vi "arduino sensirion read to stream and log (sub-vi).vi"(0 "logfile refnum":refnum<file>, 1 "VISA resource name (COM3)":refnum<visa-resource-name>="COM3", 2 "stop channel":T1, 5 "read byte count (512)":u32=512, 7 "expected num sensors (12)":i32=12, 9 "baud rate (576000)":u32=576000, 11 "error in (no error)":errorcluster) -> (8 "sensor data cluster channel":T2, 15 "error out":errorcluster)   [LabVIEW 2021]
uses:
  <extravilib>/ChannelInstances/Stream-t'sensirion_data_with_time.ctl'/)Channel.ctl
  type-defs/sensirion_data_with_time.ctl
  controls/sensirion_flow_sensor_data.ctl
  <extravilib>/ChannelInstances/Tag-bool/))Channel.ctl
  <extravilib>/ChannelInstances/Stream-t'sensirion_data_with_time.ctl'/Read With Abort.vi
  <extravilib>/ChannelInstances/Stream-t'sensirion_data_with_time.ctl'/Write With Abort.vi
  <extravilib>/ChannelInstances/Stream-t'sensirion_data_with_time.ctl'/EndpointRead.vi
  <extravilib>/ChannelInstances/Tag-bool/Read With Abort.vi
  <extravilib>/ChannelInstances/Tag-bool/Write With Abort.vi
  <extravilib>/ChannelInstances/Stream-t'sensirion_data_with_time.ctl'/Endpoint.vi
  <vilib>/Instr/_visa.llb/VISA Configure Serial Port (Instr).vi
  <extravilib>/ChannelInstances/Tag-bool/Instantiate.vi
  <extravilib>/ChannelInstances/Stream-t'sensirion_data_with_time.ctl'/Instantiate.vi
  <extravilib>/ChannelInstances/Stream-t'sensirion_data_with_time.ctl'/)Channel.vi
  <resource>/ChannelSupport/_ChannelSupport/WaitIfNeeded.vi
  <extravilib>/ChannelInstances/Tag-bool/EndpointRead.vi
  <extravilib>/ChannelInstances/Tag-bool/Endpoint.vi
  <extravilib>/ChannelInstances/Stream-t'sensirion_data_with_time.ctl'.lvlib
  <extravilib>/ChannelInstances/Tag-bool.lvlib
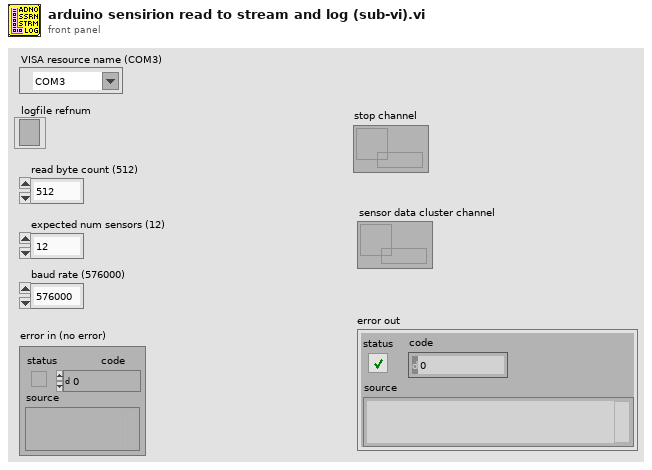
[diagram p1: front panel]
types:
  T1 = typedef "Tag-bool.lvlib/))Channel.ctl" = refnum<queue>
  T2 = typedef "Stream-t'sensirion_data_with_time.ctl'.lvlib/)Channel.ctl" = refnum<queue>
  T3 = typedef "sensirion_data_with_time.ctl" = cluster{"sensor data array":T4[], "relative timestamp":dbl, "error":errorcluster}
  T4 = typedef "sensirion_flow_sensor_data.ctl" = cluster{"flow rate \n":dbl[unit], "flow val. status":bool, "temperature":dbl[unit], "temp. val status":bool, "air in line?":bool, "high flow?":bool, "flag. val status":bool}
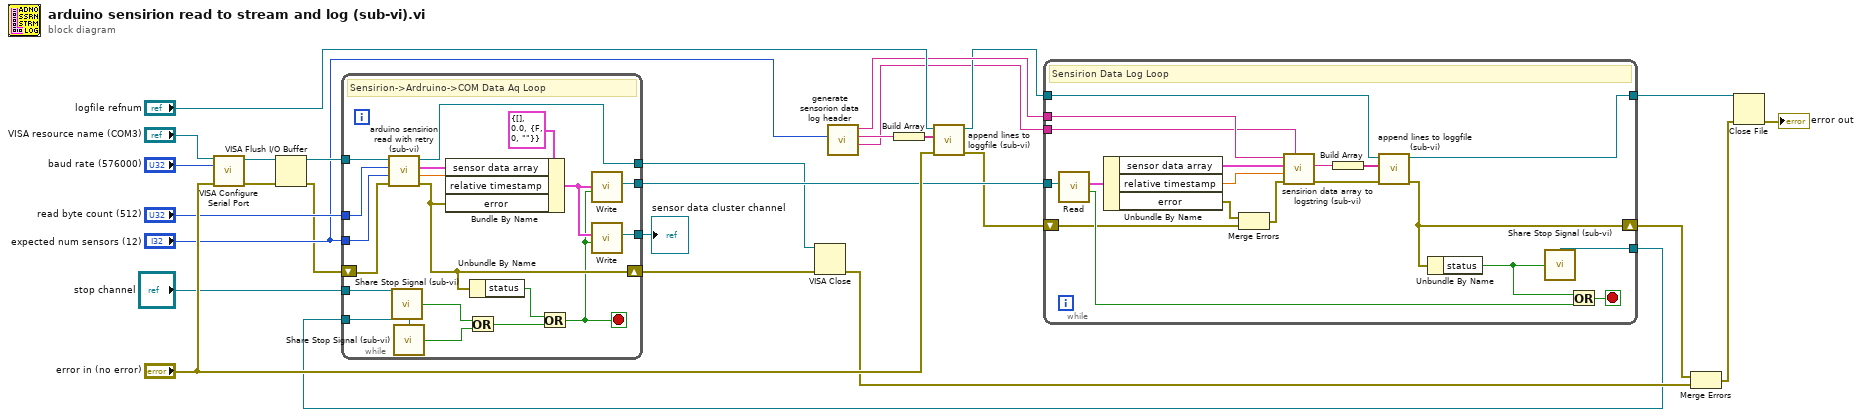
[diagram p0: block diagram]
diagram:
  n1 = call-poly "VISA Configure Serial Port"("VISA resource name"="VISA resource name (COM3)", "baud rate (9600)"="baud rate (576000)", "error in (no error)"="error in (no error)") -> ("VISA resource name out"=w23:refnum<visa-resource-name>, "error out"=w22:errorcluster)  [unwired: 11 in]
  n2 = VISA Flush I/O Buffer(VISA resource name=w23, error in (no error)=w22) -> (VISA resource name out=w18:refnum<visa-resource-name>, error out=w13:errorcluster)  [unwired: 1 in]
  n3 = call "generate sensorion data log header.vi"("num sensors"="expected num sensors (12)") -> ("delimiter"=w6:string, "sensor data header string"=w21:string, "value format"=w14:string)  [unwired: 8 in]
  n4 = Build Array(w21) -> (w20:string[])
  n5 = call "append lines to loggfile (sub-vi).vi"("error in (no error)"="error in (no error)", "string array"=w20, "file refnum"="logfile refnum") -> ("error out"=w9:errorcluster, "file refnum out"=w12:refnum<file>)  [unwired: 7 in]
  n6 = while {
    tunnel: "read byte count (512)" -> [w46]
    tunnel: w18 -> [w45]
    tunnel: [w39] -> w17
    tunnel: "expected num sensors (12)" -> [w38]
    shift-right: [w35] -> w5
    shift-left: w13 -> [w44]
    tunnel: [w37] -> w11
    tunnel: "stop channel" -> [w36]
    tunnel: [w32] -> w3
    tunnel: w1 -> [w31]
    stop <- w33 stop-if-true
    # "Sensirion->Ardruino->COM Data Aq Loop"
    n7 = call "arduino sensirion read with retry (sub-vi).vi"("error in (no error)"=w44, "expected num sensors (12)"=w38, "read byte count (512)"=w46, "VISA resource name"=w45) -> ("error out"=w35:errorcluster, "relative timestamp"=w41:dbl, "sensor data array"=w42:T4[], "VISA resource name out"=w32:refnum<visa-resource-name>)  [unwired: 3 in, 1 out]
    n8 = call "Share Stop Signal (sub-vi).vi"("channel"=w36) -> ("stop"=w30:bool)  [unwired: 1 in]
    n9 = call "Share Stop Signal (sub-vi).vi"("channel"=w31) -> ("stop"=w28:bool)  [unwired: 1 in]
    n10 = Bundle By Name(cluster=T3 {"sensor data array"=[], "relative timestamp"=0.0, "error"={"status"=FALSE, "code"=0, "source"=""}} ("Cluster"), "sensor data array"=w42, "relative timestamp"=w41, "error"=w35) -> (w40:T3)
    n11 = Or(x=w30, y=w28) -> (x .or. y?=w29:bool)
    n12 = Unbundle By Name(w35) -> ("status"=w34:bool)
    n13 = Or(x=w34, y=w29) -> (x .or. y?=w33:bool)
    n14 = call <extravilib>:"Write.vi"("last element? (F)"=w33, "element"=w40) -> ("channel"=w39:T2)  [unwired: 7 in, 2 out]
    n15 = call <extravilib>:"Write.vi"("last element? (F)"=w33, "element"=w40) -> ("channel"=w37:T2)  [unwired: 7 in, 2 out]
  }
  "sensor data cluster channel" <- w11
  n16 = VISA Close(VISA resource name=w3, error in (no error)=w5) -> (error out=w4:errorcluster)
  n17 = while {
    tunnel: w17 -> [w65]
    tunnel: w14 -> [w63]
    shift-right: [w54] -> w8
    shift-left: w9 -> [w53]
    tunnel: [w49] -> w1
    tunnel: w6 -> [w48]
    tunnel: w12 -> [w62]
    tunnel: [w57] -> w10
    stop <- w55 stop-if-true
    # "Sensirion Data Log Loop"
    n18 = call <extravilib>:"Read.vi"("channel"=w65) -> ("last element?"=w56:bool, "element"=w64:T3)  [unwired: 6 in, 3 out]
    n19 = Unbundle By Name(w64) -> ("sensor data array"=w47:T4[], "relative timestamp"=w61:dbl, "error"=w52:errorcluster)
    n20 = Merge Errors(w52, w53) -> (w51:errorcluster)
    n21 = call "sensirion data array to logstring (sub-vi).vi"("delimeter (comma)"=w48, "error in"=w51, "timestamp in relative seconds"=w61, "sensor data array"=w47, "value format (%15s)"=w63) -> ("error out"=w60:errorcluster, "string out"=w58:string)  [unwired: 5 in]
    n22 = Build Array(w58) -> (w59:string[])
    n23 = call "append lines to loggfile (sub-vi).vi"("error in (no error)"=w60, "string array"=w59, "file refnum"=w62) -> ("error out"=w54:errorcluster, "file refnum out"=w57:refnum<file>)  [unwired: 7 in]
    n24 = Unbundle By Name(w54) -> ("status"=w50:bool)
    n25 = call "Share Stop Signal (sub-vi).vi"("set stop (F)"=w50, "channel"=w49) -> ()  [unwired: 1 out]
    n26 = Or(x=w50, y=w56) -> (x .or. y?=w55:bool)
  }
  n27 = Merge Errors(w8, w4) -> (w7:errorcluster)
  n28 = Close File(refnum=w10, error in=w7) -> (error out=→"error out":errorcluster)  [unwired: 1 out]
